vi "Check Working Directory is Valid.vi"(8 "error in":errorcluster, 10 "Element to show log for":string, 11 "Working directory":path) -> (0 "error out":errorcluster, 1 "Valid?":bool)   [LabVIEW 2018, in "TortoiseGit Show Log.lvlib"]
doc: "Checks that the Working Directory is a path. Shows a dialogue and clears error if it isn't, because instead we will try to use the folder."
uses:
  TortoiseGit Show Log.lvlib
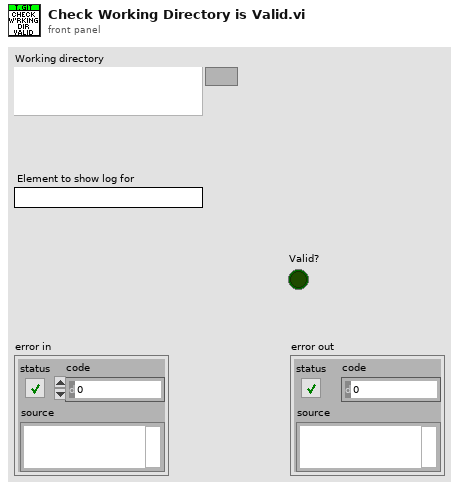
[diagram p1: front panel]
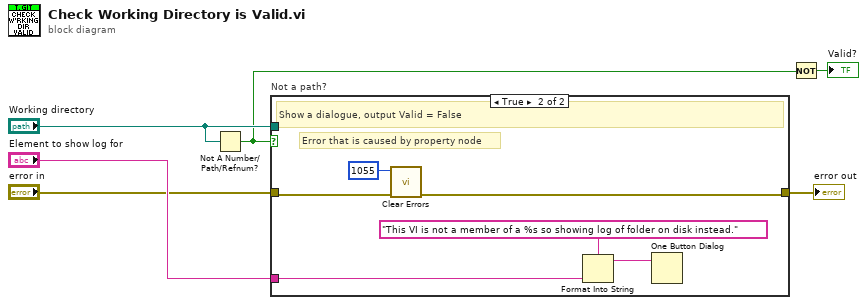
[diagram p0: block diagram]
diagram:
  n1 = Not A Number/Path/Refnum?(number/path/refnum="Working directory") -> (NaN/Path/Refnum?=w1:bool)
  n2 = case "Not a path?" shown="True" w1 {
    tunnel: [w7 w8] -> w6
    tunnel: "Working directory" -> [_ _]
    tunnel: "error in" -> [w7 w13]
    tunnel: "Element to show log for" -> [_ w10]
    frame False {
      # "VI is a path: no need to error"
    }
    frame True {
      # "Error that is caused by property node"
      # "Show a dialogue, output Valid = False"
      n3 = call <vilib>:"Clear Errors.vi"("error in (no error)"=w13, "specific error code to clear (0: all)"=1055 ("y")) -> ("error out"=w8:errorcluster)  [unwired: 4 in, 1 out]
      n4 = Format Into String(format string="This VI is not a member of a %s so showing log of folder on disk instead.", w10) -> (resulting string=w9:string)  [unwired: 2 in, 1 out]
      n5 = One Button Dialog(message=w9) -> ()  [unwired: 1 in, 1 out]
    }
  }
  "error out" <- w6
  n6 = Not(x=w1) -> (.not. x?=→"Valid?":bool)
